vi "欧姆龙PLC通讯Main-UDP.vi"(7 "拍照结果":bool=TRUE, 8 "错误in":errorcluster, 10 "写入数据":dbl[](array[numeric]), 11 "欧姆龙PLC Action":T1=enum."初始化") -> (0 "错误out":errorcluster, 3 "PLC连线成功":bool, 5 "解码成U16数组":u16[](array[numeric]))   [LabVIEW 2014]
uses:
  Controls/MsgAction.ctl
  Global.vi
panel:
  out "发送命令字符串 2":string
  out "连接的字符串":string
  out "接收数据":string
  out "打开UDP连接成功":bool
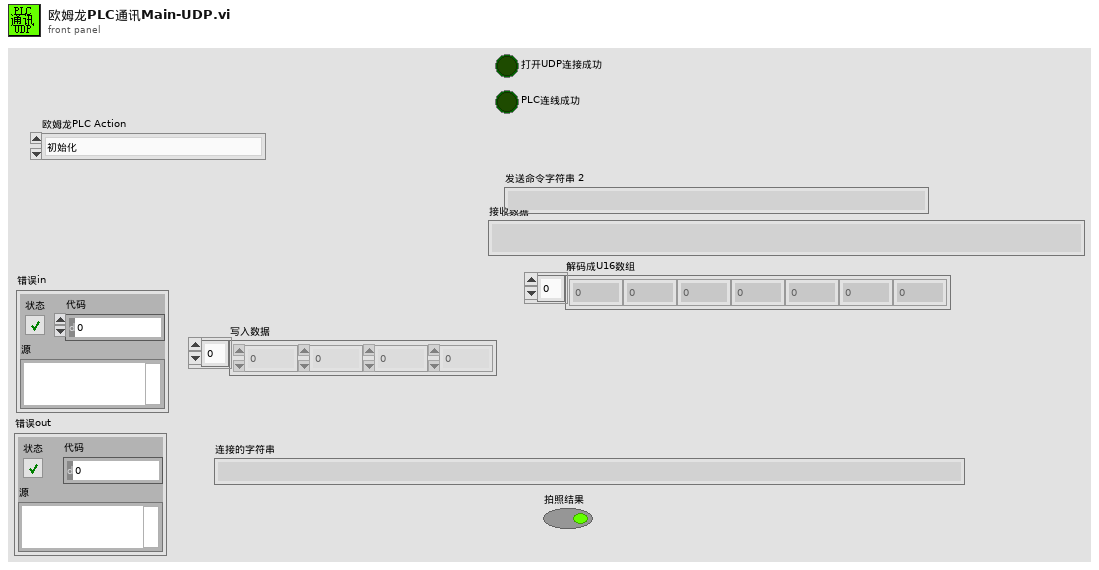
[diagram p1: front panel]
types:
  T1 = typedef "欧姆龙PLC Action.ctl" = enum16{"读设备状态", "初始化", "待命", "重新初始化", "读触发信息", "读第1组Mark点坐标", "读第2组Mark点坐标", "写基本信息", "写第1组Mark点坐标", "写第2组Mark点坐标", "写相机中心到出线头的距离", "写一笔轨迹到PLC", "写入进线前段点位", "写入板内布线点位", "写入出线布线点位", "写入数据写入完成信号", "获取信息", "写入进出线方向", "写加工信号"}
  T2 = typedef "MsgAction.ctl" = enum16{"初始化", "添加消息", "区分结果添加消息", "清空消息", "获取消息"}
  T3 = typedef "控件-UDP解码类型.ctl" = enum16{"解码Mark点号和触发信号", "解码Mark点坐标"}
  T4 = typedef "XYPos.ctl" = cluster{"X":dbl, "Y":dbl}
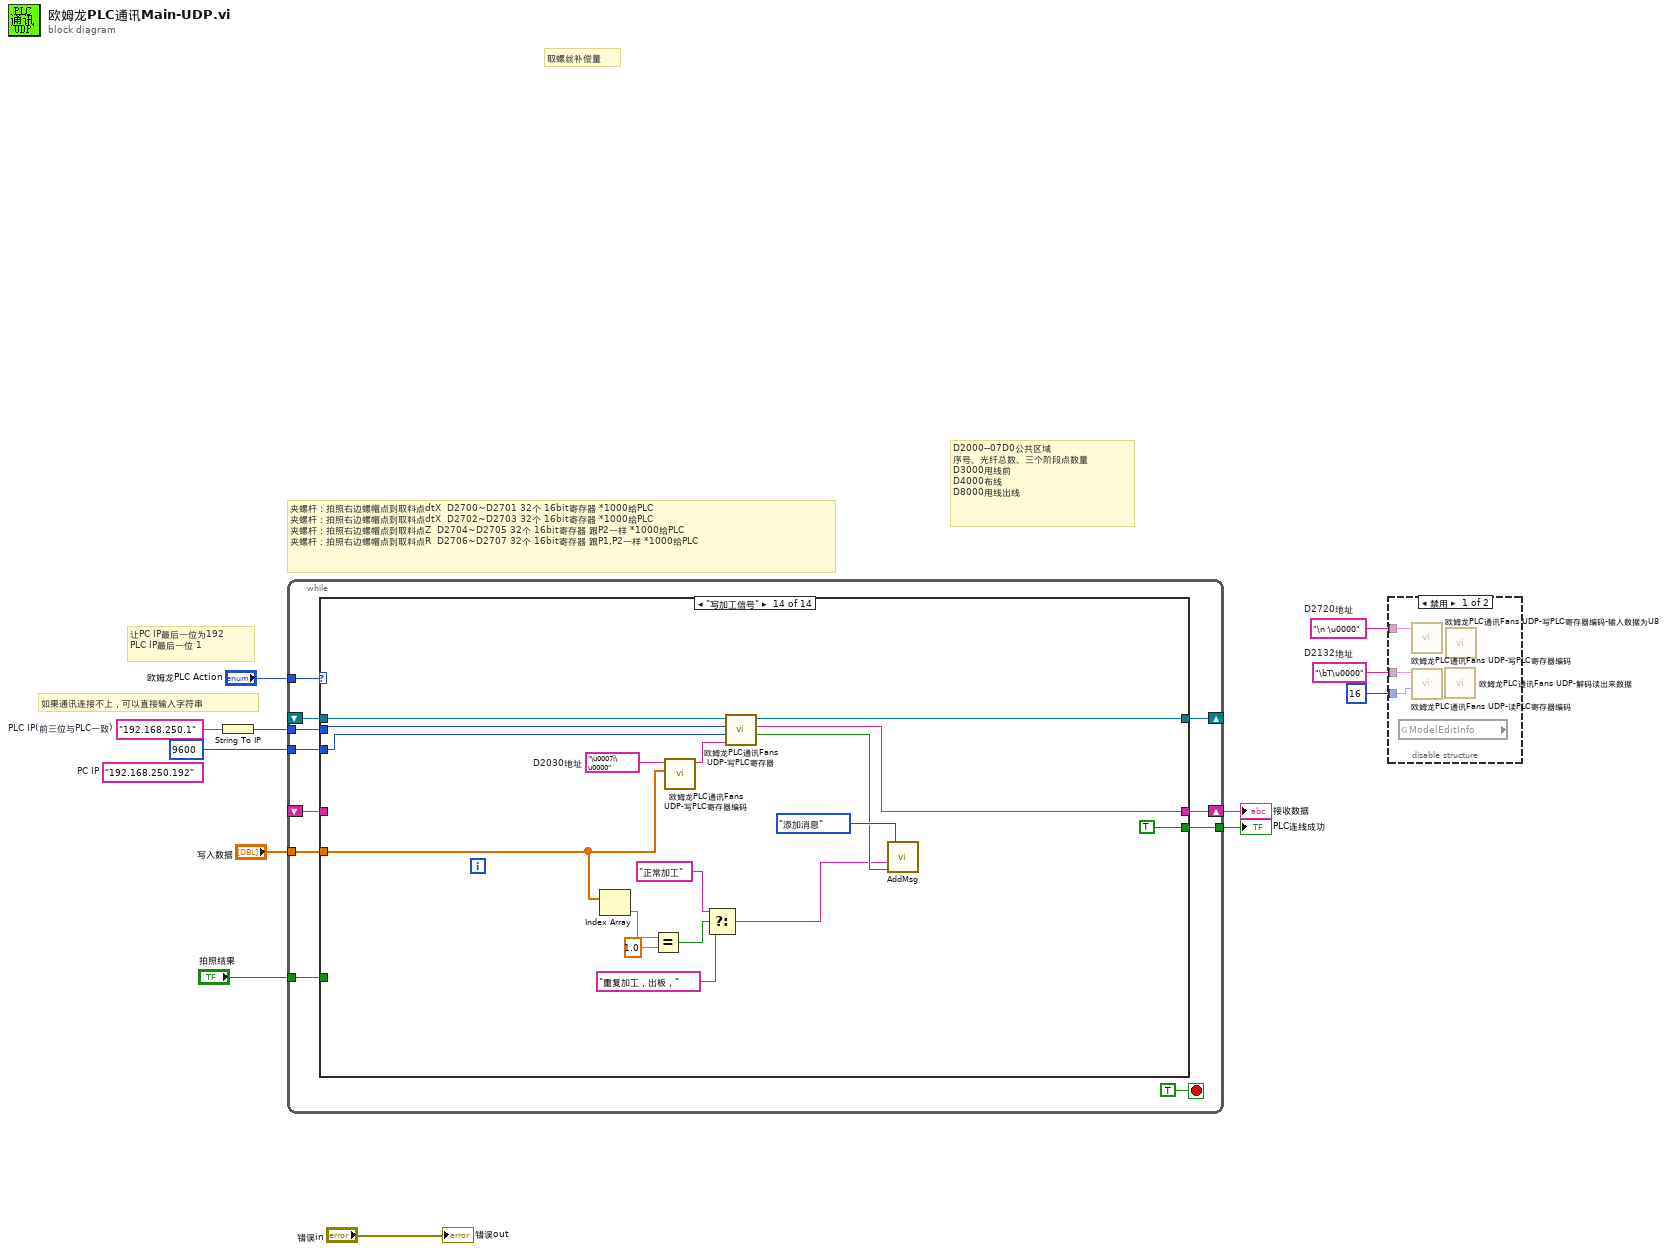
[diagram p0: block diagram]
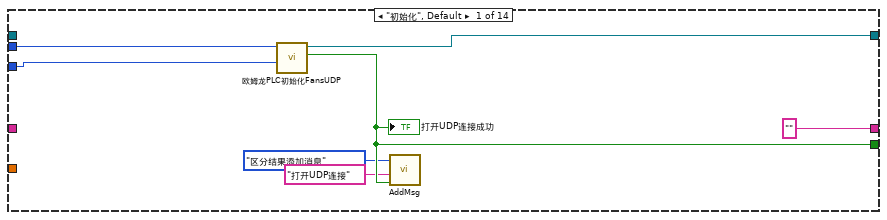
[diagram p3: hidden frame]
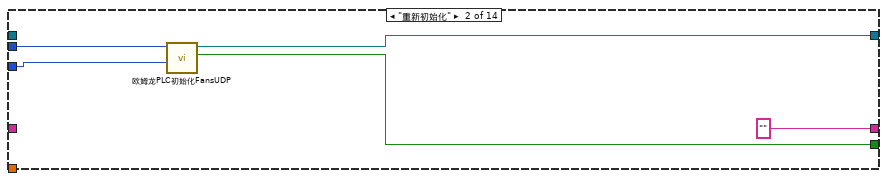
[diagram p4: hidden frame]
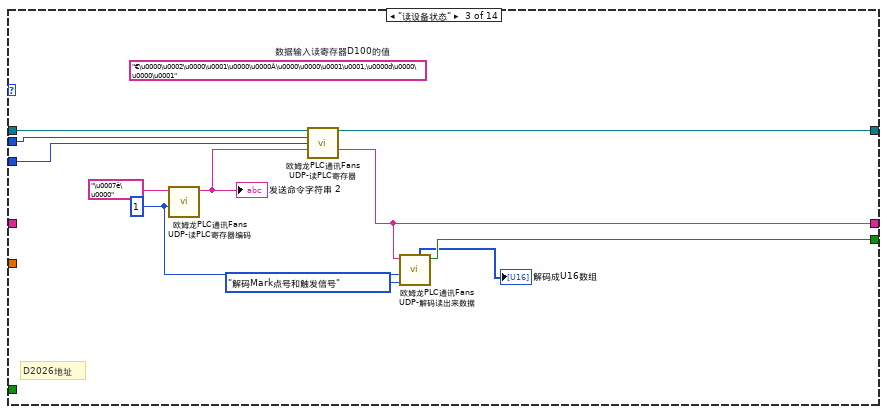
[diagram p5: hidden frame]
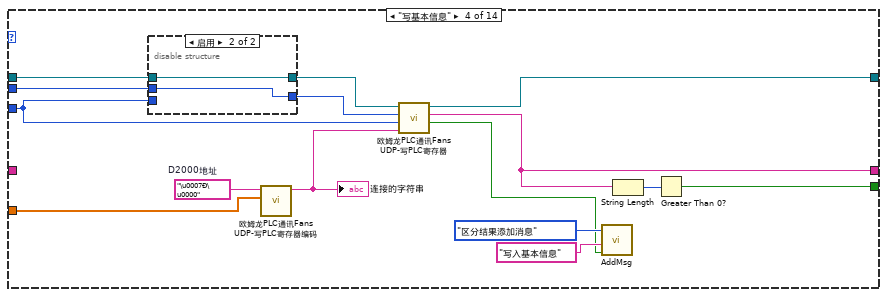
[diagram p6: hidden frame]
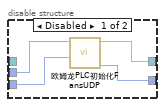
[diagram p7: hidden frame]
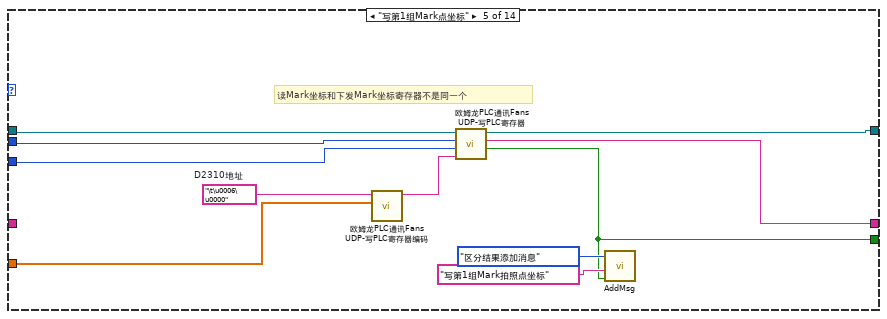
[diagram p8: hidden frame]
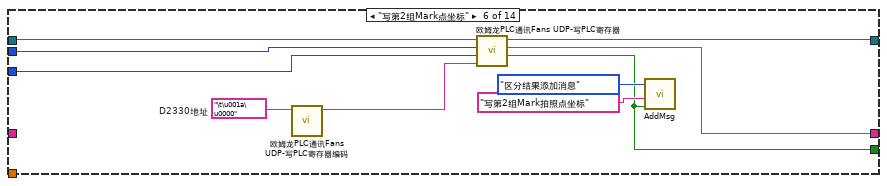
[diagram p9: hidden frame]
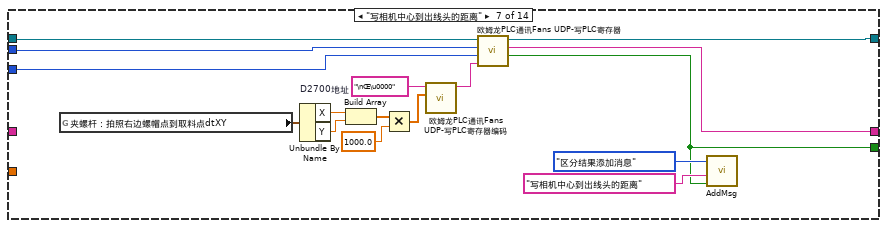
[diagram p10: hidden frame]
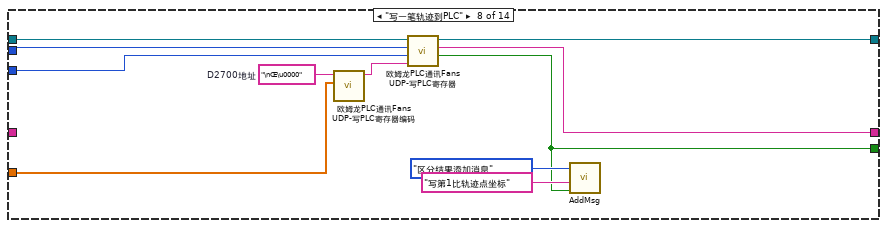
[diagram p11: hidden frame]
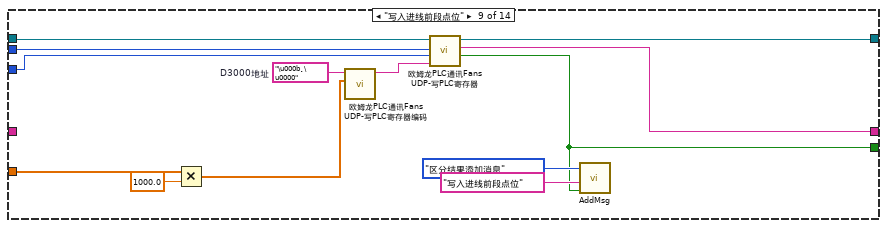
[diagram p12: hidden frame]
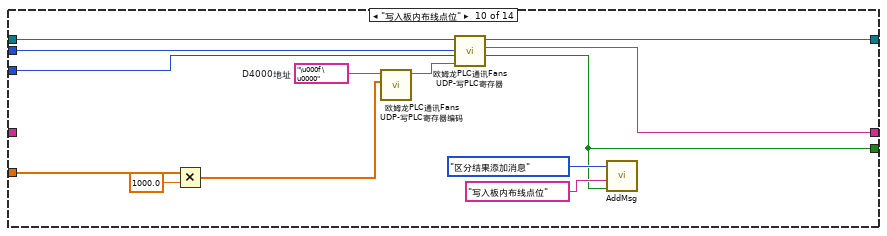
[diagram p13: hidden frame]
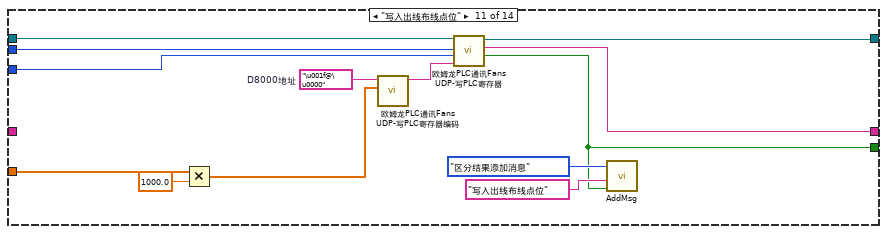
[diagram p14: hidden frame]
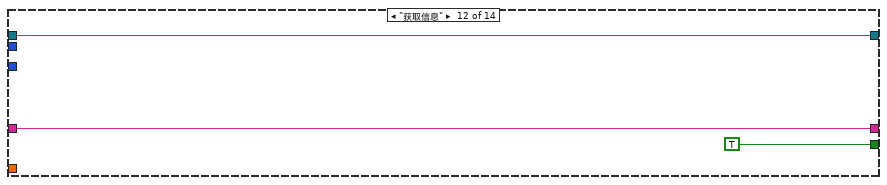
[diagram p15: hidden frame]
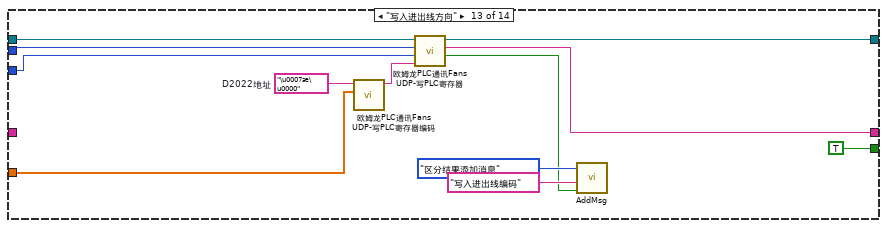
[diagram p16: hidden frame]
diagram:
  w2 = "\bT\u0000"  # D2132地址
  w3 = "\n \u0000"  # D2720地址
  (unwired) "192.168.250.192"  # PC IP
  w7 = "192.168.250.1"  # PLC IP(前三位与PLC一致)
  # "D2000--07D0公共区域\n序号、光纤总数、三个阶段点数量\nD3000甩线前\nD4000布线\nD8000甩线出线"
  # "夹螺杆：拍照右边螺帽点到取料点dtX\t\tD2700~D2701\t32个 16bit寄存器\t*1000给PLC\n夹螺杆：拍照右边螺帽点到取料点dtX\t\tD2702~D2703\t32个 16bit寄存器\t*1000给PLC\n夹螺杆：拍照右边螺帽点到取料点Z\t\tD2704~D2705\t32个 16bit寄存器\t跟P2一样 *1000给PLC\n夹螺杆：拍照右边螺帽点到取料点R\t\tD2706~D2707\t32个 16bit寄存器\t跟P1,P2一样 *1000给PLC"
  # "如果通讯连接不上，可以直接输入字符串"
  # "让PC IP最后一位为192\nPLC IP最后一位 1"
  # "取螺丝补偿量"
  n1 = String To IP(1:w7) -> (0:w6:u32)
  n2 = while {
    tunnel: "欧姆龙PLC Action" -> [w22]
    shift-right: [w21] -> _
    shift-left: _ -> [w20]
    shift-right: [w19] -> w11
    shift-left: _ -> [w18]
    tunnel: [w17] -> w10
    tunnel: "写入数据" -> [w16]
    tunnel: w6 -> [w15]
    tunnel: u16 9600 ("端口Port") -> [w14]
    tunnel: "拍照结果" -> [w13]
    stop <- TRUE ("停止") stop-if-true
    n3 = case shown="\"写加工信号\"" w22 {
      tunnel: [w27 w33 w41 w50 w73 w81 w95 w109 w120 w136 w149 w157 w165 w183] -> w21
      tunnel: w20 -> [_ _ w46 w57 w74 w84 w100 w112 w123 w137 w150 w157 w166 w184]
      tunnel: ["" ("data out") "" ("data out") w40 w51 w72 w80 w97 w108 w121 w133 w148 w156 w164 w182] -> w19
      tunnel: w18 -> [_ _ _ _ _ _ _ _ _ _ _ w156 _ _]
      tunnel: [w26 w32 w39 w59 w69 w79 w96 w105 w119 w132 w147 TRUE ("布尔") TRUE ("布尔") TRUE ("布尔")] -> w17
      tunnel: w16 -> [_ _ _ w61 w68 _ _ w106 w118 w130 w143 _ w160 w176]
      tunnel: w15 -> [w29 w34 w44 w60 w70 w83 w99 w111 w124 w135 w146 _ w159 w178]
      tunnel: w14 -> [w28 w31 w43 w53 w71 w82 w98 w110 w122 w134 w145 _ w158 w177]
      tunnel: w13 -> [_ _ _ _ _ _ _ _ _ _ _ _ _ _]
      frame "初始化", Default {
        n4 = call "欧姆龙PLC初始化FansUDP.vi"("端口Port"=w28, "PC网络地址 in"=w29) -> ("PLC初始化结果"=w26:bool, "连接ID"=w27:refnum<k16>)  [unwired: 7 in, 1 out]
        "打开UDP连接成功" <- w26
        n5 = call "AddMsg.vi"("Result"=w26, "添加消息"="打开UDP连接" ("消息显示"), "消息Action"=MsgAction."区分结果添加消息") -> ()  [unwired: 1 in, 1 out]
      }
      frame "重新初始化" {
        n6 = call "欧姆龙PLC初始化FansUDP.vi"("端口Port"=w31, "PC网络地址 in"=w34) -> ("PLC初始化结果"=w32:bool, "连接ID"=w33:refnum<k16>)  [unwired: 7 in, 1 out]
      }
      frame "读设备状态" {
        w38 = u16 1 ("读取寄存器个数")
        (unwired) "€\u0000\u0002\u0000\u0001\u0000\u0000À\u0000\u0000\u0001\u0001‚\u0000d\u0000\u0000\u0001"  # 数据输入读寄存器D100的值
        # "D2026地址"
        n7 = call "欧姆龙PLC通讯Fans UDP-读PLC寄存器编码.vi"("读取寄存器个数"=w38, "起始地址16"="\u0007ê\u0000" ("起始地址 2")) -> ("读PLC寄存器编码字符串"=w42:string)  [unwired: 9 in]
        "发送命令字符串 2" <- w42
        n8 = call "欧姆龙PLC通讯Fans UDP-读PLC寄存器.vi"("UDP网络连接输入"=w46, "IP"=w44, "端口Port"=w43, "读PLC寄存器编码字符串"=w42) -> ("UDP网络连接输出"=w41:refnum<k16>, "data out"=w40:string)  [unwired: 9 in, 1 out]
        n9 = call "欧姆龙PLC通讯Fans UDP-解码读出来数据.vi"("解码类型"=控件-UDP解码类型."解码Mark点号和触发信号", "16bit寄存器个数"=w38, "PLCoutput"=w40) -> ("回传数据长度大于0"=w39:bool, "解码成U16数组"=→"解码成U16数组":u16[])  [unwired: 4 in, 3 out]
      }
      frame "写基本信息" {
        w56 = "\u0007Ð\u0000"  # D2000地址
        n10 = disable-structure shown="启用" {
          disable-tunnel: w60 -> [w65 w66]
          disable-tunnel: w53 -> [w64 _]
          disable-tunnel: [w63 w66] -> w54
          disable-tunnel: [w62 w67] -> w55
          disable-tunnel: w57 -> [_ w67]
          frame Disabled {
            n11 = call "欧姆龙PLC初始化FansUDP.vi"("端口Port"=w64, "PC网络地址 in"=w65) -> ("网络地址"=w63:u32, "连接ID"=w62:refnum<k16>)  [unwired: 7 in, 1 out]
          }
          frame Enabled {
          }
        }
        n12 = call "欧姆龙PLC通讯Fans UDP-写PLC寄存器编码.vi"("数据"=w61, "起始地址16"=w56) -> ("写入数据编码"=w52:string)  [unwired: 9 in]
        "连接的字符串" <- w52
        n13 = call "欧姆龙PLC通讯Fans UDP-写PLC寄存器.vi"("写入数据编码"=w52, "端口Port"=w53, "IP地址"=w54, "UDP网络连接输入"=w55) -> ("布尔"=w47:bool, "data out"=w51:string, "UDP网络连接输出"=w50:refnum<k16>)  [unwired: 5 in]
        n14 = call "AddMsg.vi"("Result"=w47, "添加消息"="写入基本信息" ("消息显示"), "消息Action"=MsgAction."区分结果添加消息") -> ()  [unwired: 1 in, 1 out]
        n15 = String Length(string=w51) -> (length=w58:i32)
        n16 = Greater Than 0?(x=w58) -> (x > 0?=w59:bool)
      }
      frame "写第1组Mark点坐标" {
        w78 = "\t\u0006\u0000"  # D2310地址
        # "读Mark坐标和下发Mark坐标寄存器不是同一个"
        n17 = call "欧姆龙PLC通讯Fans UDP-写PLC寄存器编码.vi"("数据"=w68, "起始地址16"=w78) -> ("写入数据编码"=w77:string)  [unwired: 9 in]
        n18 = call "欧姆龙PLC通讯Fans UDP-写PLC寄存器.vi"("写入数据编码"=w77, "端口Port"=w71, "IP地址"=w70, "UDP网络连接输入"=w74) -> ("布尔"=w69:bool, "data out"=w72:string, "UDP网络连接输出"=w73:refnum<k16>)  [unwired: 5 in]
        n19 = call "AddMsg.vi"("Result"=w69, "添加消息"="写第1组Mark拍照点坐标" ("消息显示"), "消息Action"=MsgAction."区分结果添加消息") -> ()  [unwired: 1 in, 1 out]
      }
      frame "写第2组Mark点坐标" {
        w88 = "\t\u001a\u0000"  # D2330地址
        n20 = call "欧姆龙PLC通讯Fans UDP-写PLC寄存器编码.vi"("起始地址16"=w88) -> ("写入数据编码"=w87:string)  [unwired: 10 in]
        n21 = call "欧姆龙PLC通讯Fans UDP-写PLC寄存器.vi"("写入数据编码"=w87, "端口Port"=w82, "IP地址"=w83, "UDP网络连接输入"=w84) -> ("布尔"=w79:bool, "data out"=w80:string, "UDP网络连接输出"=w81:refnum<k16>)  [unwired: 5 in]
        n22 = call "AddMsg.vi"("Result"=w79, "添加消息"="写第2组Mark拍照点坐标" ("消息显示"), "消息Action"=MsgAction."区分结果添加消息") -> ()  [unwired: 1 in, 1 out]
      }
      frame "写相机中心到出线头的距离" {
        w104 = "\nŒ\u0000"  # D2700地址
        n23 = global read "Global.vi" "夹螺杆：拍照右边螺帽点到取料点dtXY"() -> (w94:T4)
        n24 = Unbundle By Name(w94) -> ("X"=w93:dbl, "Y"=w92:dbl)
        n25 = Build Array(w93, w92) -> (w91:dbl[])
        n26 = Multiply(x=w91, y=1000.0) -> (x*y=w89:dbl[])
        n27 = call "欧姆龙PLC通讯Fans UDP-写PLC寄存器编码.vi"("数据"=w89, "起始地址16"=w104) -> ("写入数据编码"=w103:string)  [unwired: 9 in]
        n28 = call "欧姆龙PLC通讯Fans UDP-写PLC寄存器.vi"("写入数据编码"=w103, "端口Port"=w98, "IP地址"=w99, "UDP网络连接输入"=w100) -> ("布尔"=w96:bool, "data out"=w97:string, "UDP网络连接输出"=w95:refnum<k16>)  [unwired: 5 in]
        n29 = call "AddMsg.vi"("Result"=w96, "添加消息"="写相机中心到出线头的距离" ("消息显示"), "消息Action"=MsgAction."区分结果添加消息") -> ()  [unwired: 1 in, 1 out]
      }
      frame "写一笔轨迹到PLC" {
        w107 = "\nŒ\u0000"  # D2700地址
        n30 = call "欧姆龙PLC通讯Fans UDP-写PLC寄存器编码.vi"("数据"=w106, "起始地址16"=w107) -> ("写入数据编码"=w115:string)  [unwired: 9 in]
        n31 = call "欧姆龙PLC通讯Fans UDP-写PLC寄存器.vi"("写入数据编码"=w115, "端口Port"=w110, "IP地址"=w111, "UDP网络连接输入"=w112) -> ("布尔"=w105:bool, "data out"=w108:string, "UDP网络连接输出"=w109:refnum<k16>)  [unwired: 5 in]
        n32 = call "AddMsg.vi"("Result"=w105, "添加消息"="写第1比轨迹点坐标" ("消息显示"), "消息Action"=MsgAction."区分结果添加消息") -> ()  [unwired: 1 in, 1 out]
      }
      frame "写入进线前段点位" {
        w125 = "\u000b¸\u0000"  # D3000地址
        n33 = Multiply(x=w118, y=1000.0) -> (x*y=w116:dbl[])
        n34 = call "欧姆龙PLC通讯Fans UDP-写PLC寄存器编码.vi"("数据"=w116, "起始地址16"=w125) -> ("写入数据编码"=w128:string)  [unwired: 9 in]
        n35 = call "欧姆龙PLC通讯Fans UDP-写PLC寄存器.vi"("写入数据编码"=w128, "端口Port"=w122, "IP地址"=w124, "UDP网络连接输入"=w123) -> ("布尔"=w119:bool, "data out"=w121:string, "UDP网络连接输出"=w120:refnum<k16>)  [unwired: 5 in]
        n36 = call "AddMsg.vi"("Result"=w119, "添加消息"="写入进线前段点位" ("消息显示"), "消息Action"=MsgAction."区分结果添加消息") -> ()  [unwired: 1 in, 1 out]
      }
      frame "写入板内布线点位" {
        w138 = "\u000f \u0000"  # D4000地址
        n37 = Multiply(x=w130, y=1000.0) -> (x*y=w129:dbl[])
        n38 = call "欧姆龙PLC通讯Fans UDP-写PLC寄存器编码.vi"("数据"=w129, "起始地址16"=w138) -> ("写入数据编码"=w141:string)  [unwired: 9 in]
        n39 = call "欧姆龙PLC通讯Fans UDP-写PLC寄存器.vi"("写入数据编码"=w141, "端口Port"=w134, "IP地址"=w135, "UDP网络连接输入"=w137) -> ("布尔"=w132:bool, "data out"=w133:string, "UDP网络连接输出"=w136:refnum<k16>)  [unwired: 5 in]
        n40 = call "AddMsg.vi"("Result"=w132, "添加消息"="写入板内布线点位" ("消息显示"), "消息Action"=MsgAction."区分结果添加消息") -> ()  [unwired: 1 in, 1 out]
      }
      frame "写入出线布线点位" {
        w151 = "\u001f@\u0000"  # D8000地址
        n41 = Multiply(x=w143, y=1000.0) -> (x*y=w142:dbl[])
        n42 = call "欧姆龙PLC通讯Fans UDP-写PLC寄存器编码.vi"("数据"=w142, "起始地址16"=w151) -> ("写入数据编码"=w154:string)  [unwired: 9 in]
        n43 = call "欧姆龙PLC通讯Fans UDP-写PLC寄存器.vi"("写入数据编码"=w154, "端口Port"=w145, "IP地址"=w146, "UDP网络连接输入"=w150) -> ("布尔"=w147:bool, "data out"=w148:string, "UDP网络连接输出"=w149:refnum<k16>)  [unwired: 5 in]
        n44 = call "AddMsg.vi"("Result"=w147, "添加消息"="写入出线布线点位" ("消息显示"), "消息Action"=MsgAction."区分结果添加消息") -> ()  [unwired: 1 in, 1 out]
      }
      frame "获取信息" {
      }
      frame "写入进出线方向" {
        w162 = "\u0007æ\u0000"  # D2022地址
        n45 = call "欧姆龙PLC通讯Fans UDP-写PLC寄存器编码.vi"("数据"=w160, "起始地址16"=w162) -> ("写入数据编码"=w161:string)  [unwired: 9 in]
        n46 = call "欧姆龙PLC通讯Fans UDP-写PLC寄存器.vi"("写入数据编码"=w161, "端口Port"=w158, "IP地址"=w159, "UDP网络连接输入"=w166) -> ("布尔"=w167:bool, "data out"=w164:string, "UDP网络连接输出"=w165:refnum<k16>)  [unwired: 5 in]
        n47 = call "AddMsg.vi"("Result"=w167, "添加消息"="写入进出线编码" ("消息显示"), "消息Action"=MsgAction."区分结果添加消息") -> ()  [unwired: 1 in, 1 out]
      }
      frame "写加工信号" {
        w180 = "\u0007î\u0000"  # D2030地址
        n48 = Index Array(array=w176) -> (element=w175:dbl)  [unwired: 1 in]
        n49 = Equal?(x=w175, y=1.0) -> (x = y?=w173:bool)
        n50 = call "欧姆龙PLC通讯Fans UDP-写PLC寄存器编码.vi"("数据"=w176, "起始地址16"=w180) -> ("写入数据编码"=w179:string)  [unwired: 9 in]
        n51 = Select(t="正常加工" ("消息显示"), s=w173, f="重复加工，出板，") -> (s? t:f=w171:string)
        n52 = call "欧姆龙PLC通讯Fans UDP-写PLC寄存器.vi"("写入数据编码"=w179, "端口Port"=w177, "IP地址"=w178, "UDP网络连接输入"=w184) -> ("布尔"=w185:bool, "data out"=w182:string, "UDP网络连接输出"=w183:refnum<k16>)  [unwired: 5 in]
        n53 = call "AddMsg.vi"("Result"=w185, "添加消息"=w171, "消息Action"=MsgAction."添加消息") -> ()  [unwired: 1 in, 1 out]
      }
    }
  }
  "接收数据" <- w11
  "PLC连线成功" <- w10
  n54 = disable-structure shown="禁用" {
    disable-tunnel: w3 -> [w189 _]
    disable-tunnel: w2 -> [w188 _]
    disable-tunnel: u16 16 ("读取寄存器个数") -> [w187 _]
    frame Disabled {
      n55 = global read "Global.vi" "ModelEditInfo"() -> ()  [unwired: 1 out]
      n56 = call "欧姆龙PLC通讯Fans UDP-写PLC寄存器编码.vi"("起始地址16"=w189) -> ()  [unwired: 10 in, 1 out]
      n57 = call "欧姆龙PLC通讯Fans UDP-读PLC寄存器编码.vi"("读取寄存器个数"=w187, "起始地址16"=w188) -> ()  [unwired: 9 in, 1 out]
      n58 = call "欧姆龙PLC通讯Fans UDP-解码读出来数据.vi"() -> ()  [unwired: 7 in, 5 out]
      n59 = call "欧姆龙PLC通讯Fans UDP-写PLC寄存器编码-输入数据为U8.vi"() -> ()  [unwired: 11 in, 1 out]
    }
    frame Enabled {
    }
  }
  "错误out" <- "错误in"
